vi "Read Unsigned Int Register.vi"(7 "PDU Address (U-Int16)":T1 items=["Setpoint"=33, "Setpoint slow"=34, "Alarm limit maximum"=3105, "Alarm limit minimum"=3106, "Alarm new setpoint"=3110, "Counter limit (UInt)"=3331, "Counter new setpoint"=3334, "Valve output"=61960], 8 "error in":errorcluster, 11 "MB_TCP session in":refnum<class "MB_Master_TCP.lvclass">) -> (0 "error out":errorcluster, 2 "Value":u16, 3 "MB session out":refnum<class "MB_Master_TCP.lvclass">)   [LabVIEW 2024, in "Bronkhorst Flexi-Flow ModbusTCP API.lvlib"]
uses:
  Bronkhorst Flexi-Flow ModbusTCP API.lvlib
  <vilib>/Plasmionique/MB Master/MB_Master_TCP/MB_Master_TCP.lvclass
  C:/Program Files/National Instruments/LabVIEW 2025/vi.lib/Plasmionique/MB Master/MB_Master/MB_Master.lvclass
  PDU Address U16 Params--ring.ctl
  <vilib>/Plasmionique/MB Master/MB Master.lvlib
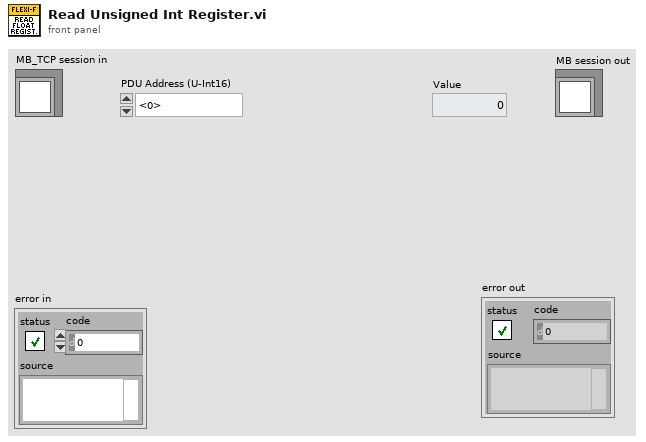
[diagram p1: front panel]
types:
  T1 = typedef "Bronkhorst Flexi-Flow ModbusTCP API.lvlib/PDU Address U16 Params--ring.ctl" = u16
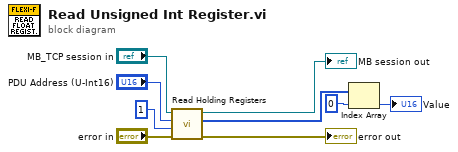
[diagram p0: block diagram]
diagram:
  n1 = call <vilib>:"Read Holding Registers.vi"("error in (no error)"="error in", "quantity"=u16 1, "starting address"="PDU Address (U-Int16)", "MB session in"="MB_TCP session in") -> ("error out"=→"error out":errorcluster, "Registers"=w3:u16[], "MB session out"=→"MB session out":refnum<class "MB_Master_TCP.lvclass">)  [unwired: 5 in]
  n2 = Index Array(array=w3, index=0) -> (element=→"Value":u16)
